vi "Write KFMParam.vi"(6 "timeouts":T2[](array[typedef]), 8 "error in (no error)":errorcluster, 9 "IP Address":T1(array[cluster]), 10 "MVIName":string[](array[string]), 11 "KFMParam in":T3) -> (0 "error out":errorcluster, 3 "KFMParam out":T3)   [LabVIEW 2021, in "ICPCON_Param.lvlib"]
uses:
  ICPCON_Param.lvlib
  ICPCON Param.ctl
  Eth timeouts.ctl
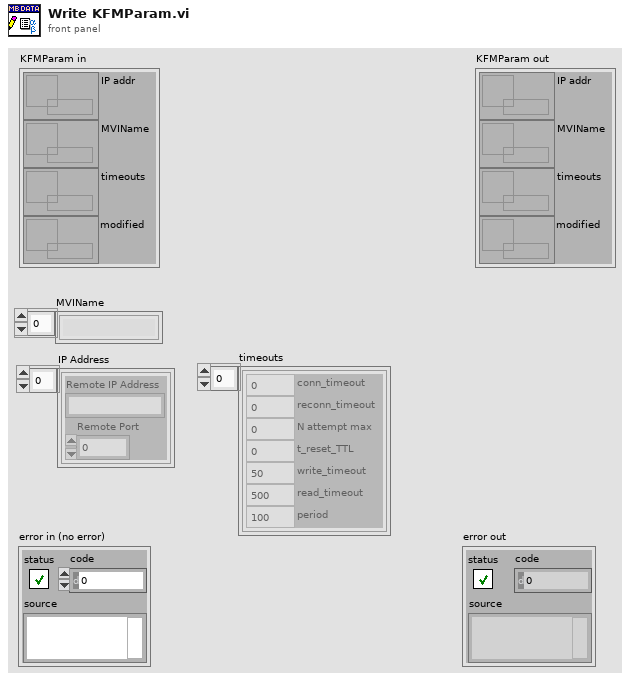
[diagram p1: front panel]
types:
  T1 = cluster{"Remote IP Address":string, "Remote Port":u16}[]
  T2 = typedef "ICPCON_Param.lvlib/Eth timeouts.ctl" = cluster{"conn_timeout":i32, "reconn_timeout":i32, "N attempt max":i32, "t_reset_TTL":i32, "write_timeout":i32, "read_timeout":i32, "period":i32}
  T3 = typedef "ICPCON_Param.lvlib/ICPCON Param.ctl" = cluster{"IP addr":refnum<data-value>, "MVIName":refnum<data-value>, "timeouts":refnum<data-value>, "modified":refnum<data-value>}
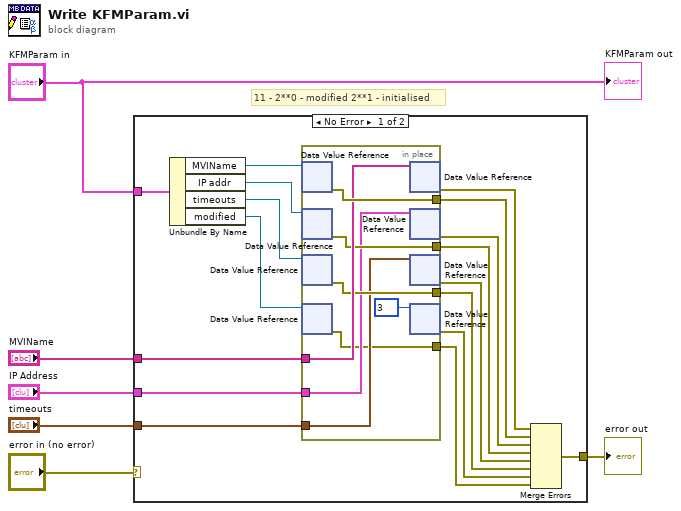
[diagram p0: block diagram]
diagram:
  # "11 - 2**0 - modified 2**1 - initialised"
  n1 = case shown="No Error" "error in (no error)" {
    selector: "error in (no error)" -> [_ w32]
    tunnel: [w21 w32] -> w5
    tunnel: "KFMParam in" -> [w20 _]
    tunnel: "MVIName" -> [w19 _]
    tunnel: "IP Address" -> [w18 _]
    tunnel: "timeouts" -> [w17 _]
    frame No Error {
      n2 = Unbundle By Name(w20) -> ("MVIName"=w12:refnum<data-value>, "IP addr"=w11:refnum<data-value>, "timeouts"=w10:refnum<data-value>, "modified"=w9:refnum<data-value>)
      n3 = in-place {
        in-place-border: [w31] -> w22
        in-place-border: w19 -> [w30]
        in-place-border: [w29] -> w15
        in-place-border: [w28] -> w13
        in-place-border: w18 -> [w27]
        in-place-border: w17 -> [w26]
        in-place-border: [w24] -> w7
        n4 = in-place-dvr #1(w12) -> (w31:errorcluster)  [unwired: 1 out]
        n5 = in-place-dvr #2(w11) -> (w29:errorcluster)  [unwired: 1 out]
        n6 = in-place-dvr #3(w10) -> (w28:errorcluster)  [unwired: 1 out]
        n7 = in-place-dvr #4(w9) -> (w24:errorcluster)  [unwired: 1 out]
        n8 = in-place-dvr #1(w30) -> (w23:errorcluster)  [unwired: 1 out]
        n9 = in-place-dvr #2(w27) -> (w16:errorcluster)  [unwired: 1 out]
        n10 = in-place-dvr #3(w26) -> (w14:errorcluster)  [unwired: 1 out]
        n11 = in-place-dvr #4(u8 3 ("data value")) -> (w8:errorcluster)  [unwired: 1 out]
      }
      n12 = Merge Errors(w23, w22, w16, w15, w14, w13, w8, w7) -> (w21:errorcluster)
    }
    frame Error {
    }
  }
  "error out" <- w5
  "KFMParam out" <- "KFMParam in"
